vi "ACT_limit_setpoint_and_control_internal.vi"(0 "MD420.lvclass":refnum<class "MD420.lvclass">, 1 "PG < 10%":bool, 2 "PG Setpoint Min":dbl, 3 "ACT SP Ctrl":bool, 4 "ACT lower limit":dbl, 5 "ACT limit Setpoint":dbl, 6 "PG1":dbl, 7 "error in":errorcluster, 8 "PG target Setpoint":dbl) -> (20 "MD420.lvclass out":refnum<class "MD420.lvclass">, 22 "Increase ACT\nlimit Setpoint":bool, 24 "ACT SP Ctrl\nOFF":bool, 27 "error out":errorcluster)   [LabVIEW 2022 SP3, in "MD420.lvclass"]
uses:
  MD420.lvclass
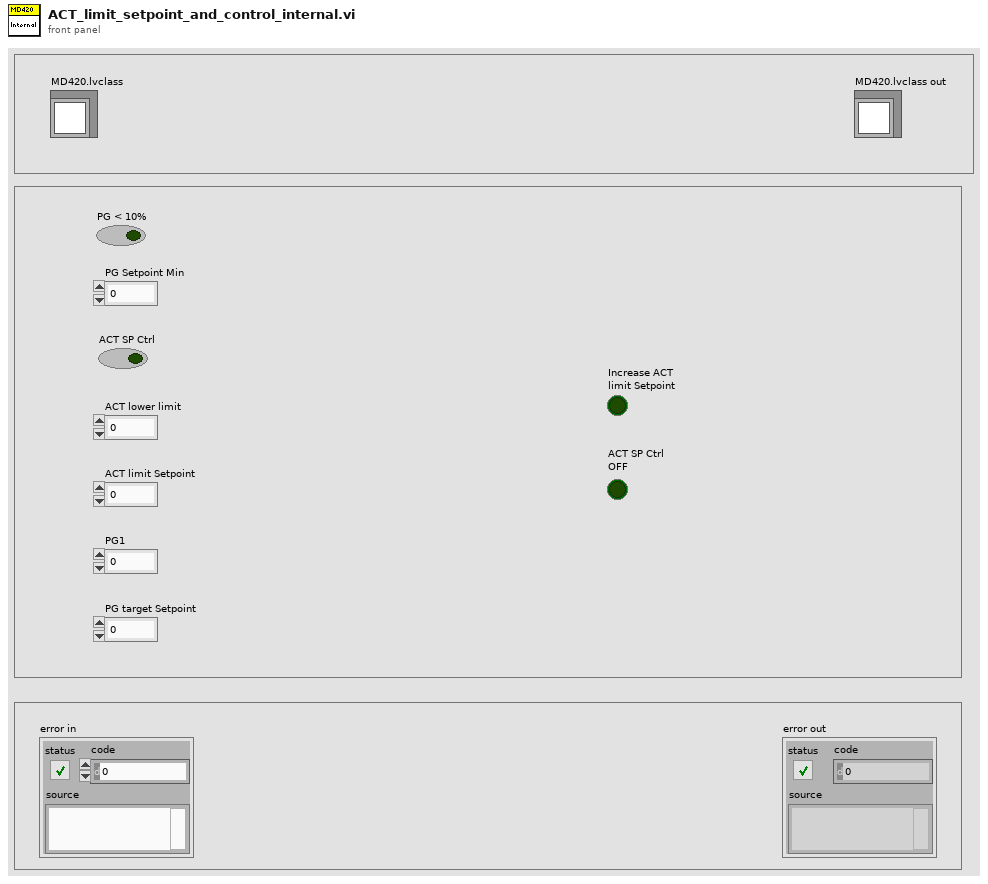
[diagram p1: front panel]
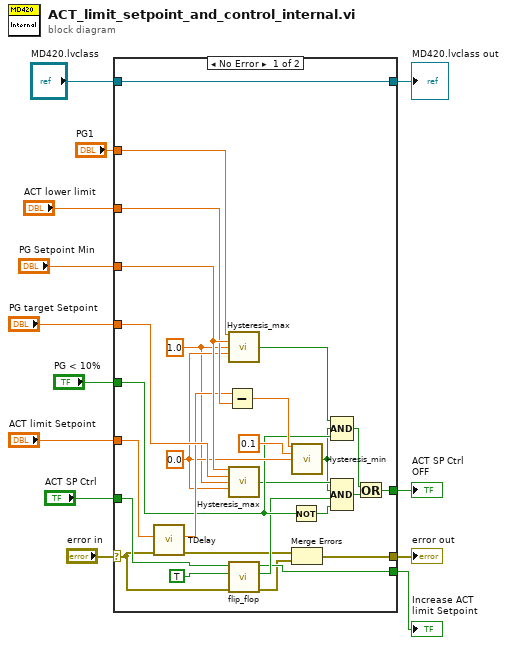
[diagram p0: block diagram]
diagram:
  n1 = case shown="No Error" "error in" {
    selector: "error in" -> [w18 w42]
    tunnel: "PG Setpoint Min" -> [w38 _]
    tunnel: "PG1" -> [w39 _]
    tunnel: "PG target Setpoint" -> [w37 _]
    tunnel: "ACT lower limit" -> [w35 _]
    tunnel: "ACT limit Setpoint" -> [w34 _]
    tunnel: "ACT SP Ctrl" -> [w40 _]
    tunnel: "PG < 10%" -> [w28 _]
    tunnel: [w21 _] -> w4
    tunnel: [w20 _] -> w5
    tunnel: [w15 w42] -> w3
    tunnel: "MD420.lvclass" -> [w14 w41]
    tunnel: [w14 w41] -> w1
    frame No Error {
      w31 = 1.0 ("H")
      w32 = 0.0 ("Max")
      n2 = call "TDelay.vi"("Error in"=w18, "input"=w34) -> ("Error out"=w17:errorcluster, "output"=w33:dbl)  [unwired: 8 in]
      n3 = Subtract(x=w33, y=w35) -> (x-y=w36:dbl)
      n4 = call "Hysteresis_max.vi"("input(+)"=w39, "input (-)"=w38, "H"=w31, "Max"=w32) -> ("Deviation"=w29:bool)  [unwired: 10 in, 1 out]
      n5 = call "Hysteresis_max.vi"("input(+)"=w38, "input (-)"=w37, "H"=w31, "Max"=w32) -> ("Deviation"=w26:bool)  [unwired: 10 in, 1 out]
      n6 = call "flip_flop.vi"("error in"=w18, "BI2"=TRUE, "BI1"=w40) -> ("error out"=w16:errorcluster, "BO2"=w24:bool, "BO1"=w20:bool)  [unwired: 6 in]
      n7 = Not(x=w28) -> (.not. x?=w27:bool)
      n8 = call "Hysteresis_min.vi"("input"=w36, "Min"=0.1, "H"=w32) -> ("Deviation"=w25:bool)  [unwired: 11 in, 1 out]
      n9 = Merge Errors(w17, w16) -> (w15:errorcluster)
      n10 = Compound Arithmetic op=AND(w29, w25, w28) -> (w23:bool)
      n11 = Compound Arithmetic op=AND(w26, w25, w24, w27) -> (w22:bool)
      n12 = Or(x=w23, y=w22) -> (x .or. y?=w21:bool)
    }
    frame Error {
    }
  }
  "Increase ACT\nlimit Setpoint" <- w5
  "ACT SP Ctrl\nOFF" <- w4
  "error out" <- w3
  "MD420.lvclass out" <- w1
